vi "Chrg_Dschrg_nodaq.vi"(3 "PS type":enum16{"NHR", "ITECH"}(ring), 4 "PS VISA in":refnum<visa-resource-name>, 5 "PS error in":errorcluster caption="PS error in (no error)", 6 "CyclePath":path=path "C:/Users/ga11/Desktop/VI/results/3PtestCharge.lvm" caption="Filename", 7 "Battery Type":enum16{"30Q", "40T"}(ring), 8 "Charge/discharge":enum8{"Charge", "Discharge"}(ring), 9 "Charge/Discharge Voltage Setpoint":dbl format="%#.6g", 11 "Current Setpoint":dbl format="%#.6g", 13 "Current Cutoff":dbl) -> (14 "PS VISA out":refnum<visa-resource-name>, 19 "PS error out":errorcluster)   [LabVIEW 2020]
uses:
  Drivers-Essentials/Read (Ave Current).vi
  Drivers-NHR-9200/NHR/Public/Data/Low Level/Fetch (Ave Voltage).vi
  <vilib>/Utility/TradDaqScaling.llb/Convert Strain Gauge Reading (scaler).vi
  Drivers-Essentials/NH Research Regenerative Test Series.lvlib
  Drivers-IT-M3400/IT-M3400.lvlib
panel:
  out "StrainGauge":dbl format="%.10f"
  out "Thermocouple":dbl format="%.2f"
  out "Read Ave Current (A)":dbl
  out "Read Ave Voltage (V)":dbl
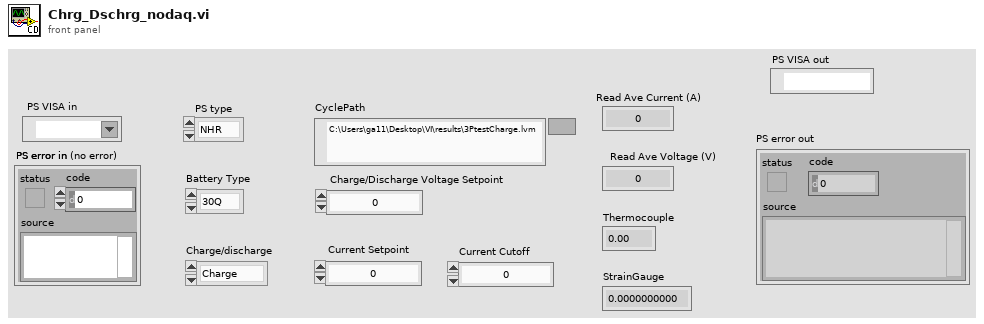
[diagram p1: front panel]
types:
  T1 = cluster{"Voltage Enabled":bool, "Current Enabled":bool, "Power Enabled":bool, "Resistance Enabled":bool}
  T2 = cluster{"Baud Rate":u32, "Parity":u16, "Data Bits":u16, "Stop Bits":u16, "Flow Control":u16}
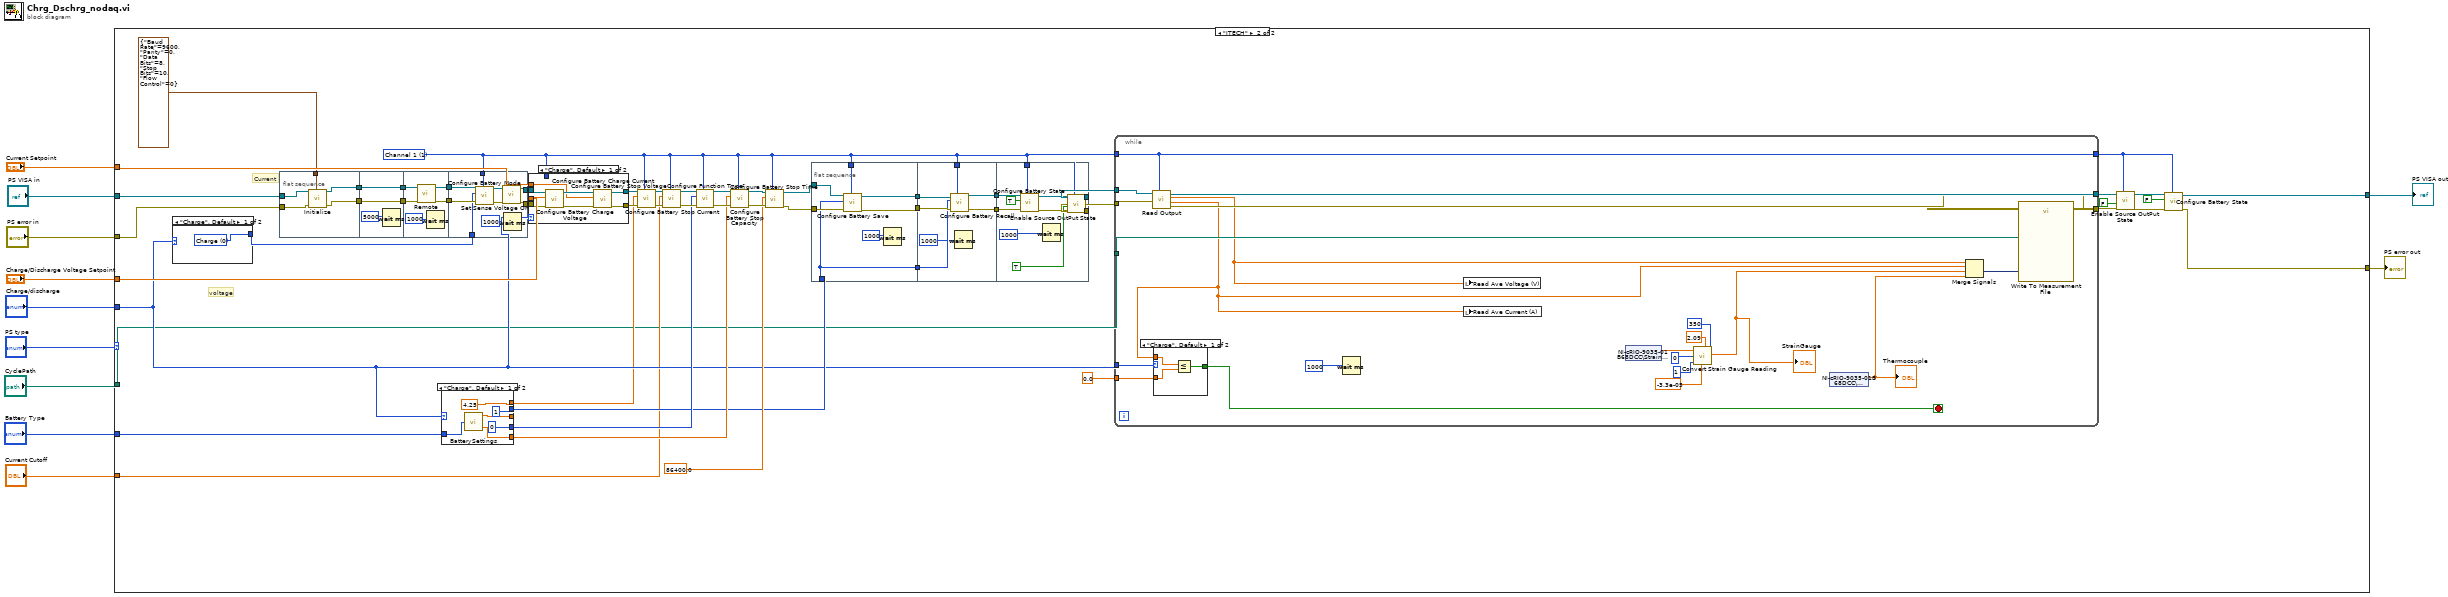
[diagram p0: block diagram]
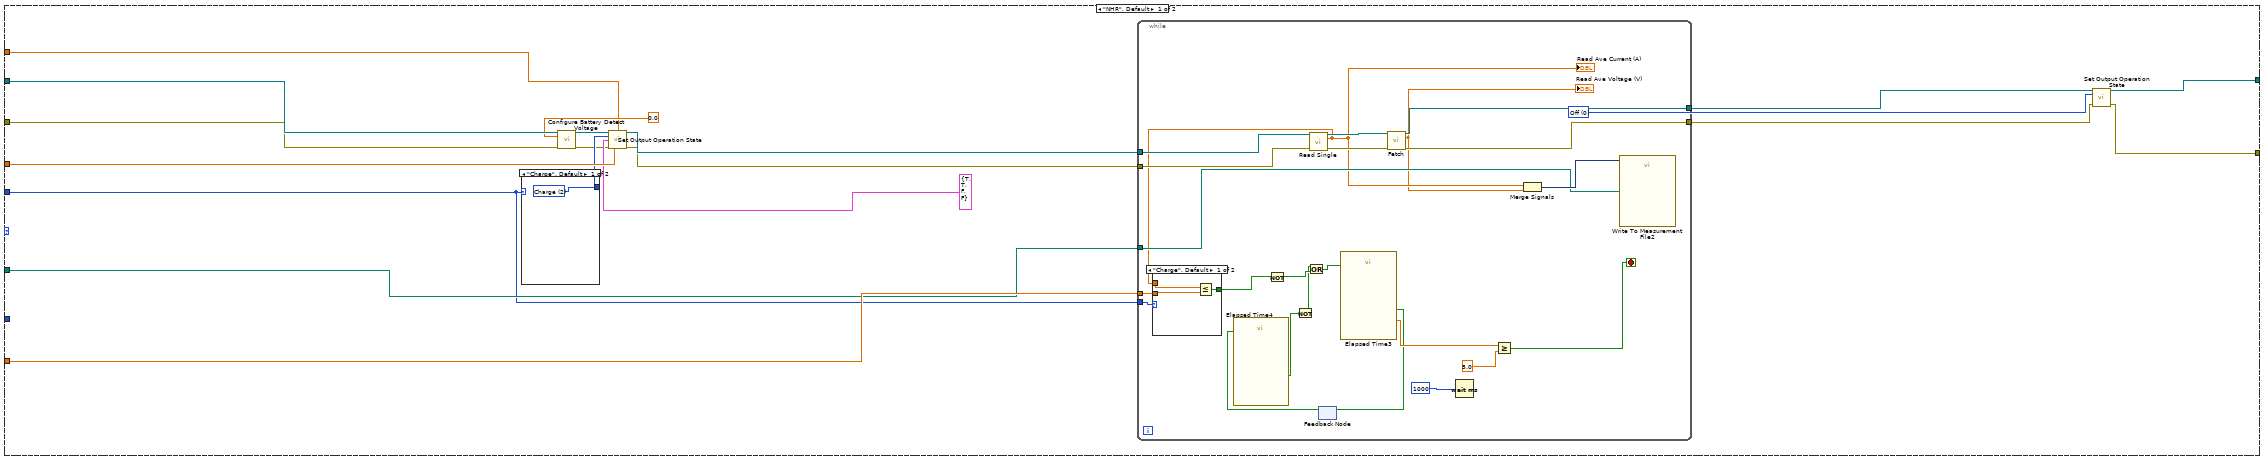
[diagram p2: hidden frame]
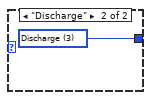
[diagram p3: hidden frame]
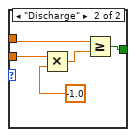
[diagram p4: hidden frame]
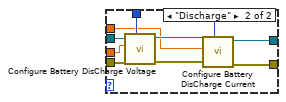
[diagram p5: hidden frame]
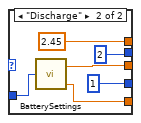
[diagram p6: hidden frame]
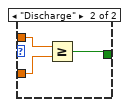
[diagram p7: hidden frame]
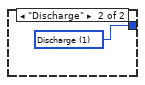
[diagram p8: hidden frame]
diagram:
  n1 = case shown="\"ITECH\"" "PS type" {
    tunnel: "Charge/Discharge Voltage Setpoint" -> [w30 w101]
    tunnel: "Current Setpoint" -> [w12 w99]
    tunnel: "Current Cutoff" -> [w27 w69]
    tunnel: "CyclePath" -> [w24 w67]
    tunnel: "PS VISA in" -> [w20 w80]
    tunnel: "PS error in" -> [w19 w79]
    tunnel: [w17 w66] -> w1
    tunnel: [w16 w100] -> w5
    tunnel: "Charge/discharge" -> [w13 w70]
    tunnel: "Battery Type" -> [_ w98]
    frame "NHR", Default {
      w23 = 0 items=["Off", "Standby", "Charge", "Discharge", "Battery"] ("Mode (0: Off)")
      n2 = case shown="\"Charge\", Default" w13 {
        tunnel: [w31 w32] -> w25
        frame "Charge", Default {
          w31 = 2 items=["Off", "Standby", "Charge", "Discharge", "Battery"] ("Mode (0: Off)")
        }
        frame "Discharge" {
          w32 = 3 items=["Off", "Standby", "Charge", "Discharge", "Battery"] ("Mode (0: Off)")
        }
      }
      n3 = call "Configure Battery Detect Voltage.vi"("VISA resource name"=w20, "Battery Detect Voltage (0V)"=0.0, "error in (no error)"=w19) -> ("VISA resource name out"=w22:refnum<visa-resource-name>, "error out"=w21:errorcluster)  [unwired: 11 in]
      n4 = call "Set Output Operation State.vi"("VISA resource name"=w22, "Voltage Setpoint (0 V)"=w30, "Current Setpoint (0 A)"=w12, "Mode (0: Off)"=w25, "Enable"=T1 {"Voltage Enabled"=TRUE, "Current Enabled"=TRUE, "Power Enabled"=FALSE, "Resistance Enabled"=FALSE}, "error in (no error)"=w21) -> ("VISA resource name out"=w29:refnum<visa-resource-name>, "error out"=w28:errorcluster)  [unwired: 8 in]
      n5 = while {
        tunnel: w29 -> [w53]
        tunnel: w28 -> [w52]
        tunnel: w27 -> [w37]
        tunnel: w24 -> [w40]
        tunnel: [w39] -> w15
        tunnel: [w38] -> w14
        tunnel: w13 -> [w36]
        stop <- w43 stop-if-true
        n6 = call-poly "Read Single.vi"("VISA resource name"=w53, "error in (no error)"=w52) -> ("VISA resource name out"=w54:refnum<visa-resource-name>, "Ave Current (A)"=w35:dbl, "error out"=w55:errorcluster)  [unwired: 11 in]
        "Read Ave Current (A)" <- w35
        n7 = case shown="\"Charge\", Default" w36 {
          tunnel: w37 -> [w57 w62]
          tunnel: w35 -> [w58 w60]
          tunnel: [w56 w59] -> w34
          frame "Charge", Default {
            n8 = Less Or Equal?(x=w58, y=w57) -> (x <= y?=w56:bool)
          }
          frame "Discharge" {
            n9 = Multiply(x=w62, y=-1.0) -> (x*y=w61:dbl)
            n10 = Greater Or Equal?(x=w60, y=w61) -> (x >= y?=w59:bool)
          }
        }
        n11 = Not(x=w34) -> (.not. x?=w49:bool)
        n12 = feedback #1() -> (w41:bool)  [unwired: 1 in]
        n13 = call "Elapsed Time4"("Reset"=w41) -> ("Time has Elapsed"=w48:bool)  [unwired: 11 in, 7 out]
        n14 = Not(x=w48) -> (.not. x?=w47:bool)
        n15 = Or(x=w47, y=w49) -> (x .or. y?=w46:bool)
        n16 = call "Elapsed Time3"("Reset"=w46) -> ("Elapsed Time (s)"=w45:dbl, "Time has Elapsed"=w42:bool)  [unwired: 11 in, 6 out]
        n17 = feedback-in #1(w42) -> ()
        n18 = call-poly "Fetch.vi"("VISA resource name"=w54, "error in (no error)"=w55) -> ("VISA resource name out"=w39:refnum<visa-resource-name>, "Ave Voltage (V)"=w33:dbl, "error out"=w38:errorcluster)  [unwired: 11 in]
        "Read Ave Voltage (V)" <- w33
        n19 = Wait (ms)(milliseconds to wait=1000) -> ()  [unwired: 1 out]
        n20 = Greater Or Equal?(x=w45, y=5.0) -> (x >= y?=w43:bool)
        n21 = Merge Signals "Merge Signals"(w35, w33) -> (w51:dynamicdata)
        n22 = call "Write To Measurement File2"("Signals"=w51, "Filename"=w40) -> ()  [unwired: 15 in, 3 out]
      }
      n23 = call "Set Output Operation State.vi"("VISA resource name"=w15, "Mode (0: Off)"=w23, "error in (no error)"=w14) -> ("VISA resource name out"=w17:refnum<visa-resource-name>, "error out"=w16:errorcluster)  [unwired: 11 in]
    }
    frame "ITECH" {
      w72 = 1 items=["Channel 1"=1, "Channel 2"=2, "Channel 3"=3, "Channel 4"=4, "Channel 5"=5, "Channel 6"=6, "Channel 7"=7, "Channel 8"=8, "Channel 8"=9, "Channel 10"=10, "Channel 11"=11, "Channel 12"=12, "Channel 13"=13, "Channel 14"=14, "Channel 15"=15, "Channel 16"=16] ("Channel")
      # "voltage"
      # "Current"
      n24 = case shown="\"Charge\", Default" w70 {
        tunnel: [w219 w220] -> w86
        frame "Charge", Default {
          w219 = u8 0 items=["Charge", "Discharge"] ("Battery Mode")
        }
        frame "Discharge" {
          w220 = u8 1 items=["Charge", "Discharge"] ("Battery Mode")
        }
      }
      n25 = flat-sequence {
        tunnel: [w117] -> w84
        tunnel: [w118] -> w82
        tunnel: T2 {"Baud Rate"=9600, "Parity"=0, "Data Bits"=8, "Stop Bits"=10, "Flow Control"=0} ("Serial Configuration") -> [w121]
        tunnel: w79 -> [w120]
        tunnel: w80 -> [w119]
        tunnel: w84 -> [w124]
        tunnel: [w124] -> w83
        tunnel: w82 -> [w123]
        tunnel: [w123] -> w81
        tunnel: [w129] -> w88
        tunnel: [w128] -> w87
        tunnel: w83 -> [w127]
        tunnel: w81 -> [w126]
        tunnel: w88 -> [w135]
        tunnel: w87 -> [w137]
        tunnel: w72 -> [w138]
        tunnel: w86 -> [w136]
        tunnel: [w131] -> w65
        tunnel: [w130] -> w64
        frame #0 {
          n26 = call "Initialize.vi"("Serial Configuration"=w121, "error in"=w120, "VISA resource name"=w119) -> ("error out"=w118:errorcluster, "VISA resource name out"=w117:refnum<visa-resource-name>)  [unwired: 7 in]
        }
        frame #1 {
          n27 = Wait (ms)(milliseconds to wait=5000) -> ()  [unwired: 1 out]
        }
        frame #2 {
          n28 = call "Remote.vi"("error in"=w126, "VISA resource name"=w127) -> ("error out"=w128:errorcluster, "VISA resource name out"=w129:refnum<visa-resource-name>)  [unwired: 8 in]
          n29 = Wait (ms)(milliseconds to wait=1000) -> ()  [unwired: 1 out]
        }
        frame #3 {
          n30 = call "Configure Battery Mode.vi"("Channel"=w138, "error in"=w137, "Battery Mode"=w136, "VISA resource name"=w135) -> ("error out"=w132:errorcluster, "VISA resource name out"=w133:refnum<visa-resource-name>)  [unwired: 6 in]
          n31 = call "Set Sense Voltage On.vi"("error in"=w132, "VISA resource name"=w133) -> ("error out"=w131:errorcluster, "VISA resource name out"=w130:refnum<visa-resource-name>)  [unwired: 8 in]
          n32 = Wait (ms)(milliseconds to wait=1000) -> ()  [unwired: 1 out]
        }
      }
      n33 = case shown="\"Charge\", Default" w70 {
        tunnel: w98 -> [w185 w191]
        tunnel: [w184 w189] -> _
        tunnel: [u8 0 ("File") u8 1 ("File")] -> w74
        tunnel: [u8 1 ("File") u8 2 ("File")] -> w71
        tunnel: [w181 w187] -> w73
        tunnel: [4.25 2.45] -> w68
        frame "Charge", Default {
          n34 = call "BatterySettings.vi"("Battery Type"=w185) -> ("RatedCapacity (Ah)"=w181:dbl, "Max Voltage (V)"=w184:dbl)  [unwired: 2 in, 1 out]
        }
        frame "Discharge" {
          n35 = call "BatterySettings.vi"("Battery Type"=w191) -> ("RatedCapacity (Ah)"=w187:dbl, "Min Voltage (V)"=w189:dbl)  [unwired: 2 in, 1 out]
        }
      }
      n36 = case shown="\"Charge\", Default" w70 {
        tunnel: w64 -> [w170 w179]
        tunnel: w65 -> [w169 w178]
        tunnel: [w164 w175] -> w108
        tunnel: [w163 w174] -> w107
        tunnel: w72 -> [_ w173]
        tunnel: w101 -> [w166 w172]
        tunnel: w99 -> [w165 w171]
        frame "Charge", Default {
          n37 = call "Configure Battery Charge Voltage.vi"("error in"=w169, "Charge Voltage(V)"=w166, "VISA resource name"=w170) -> ("error out"=w167:errorcluster, "VISA resource name out"=w168:refnum<visa-resource-name>)  [unwired: 6 in]
          n38 = call "Configure Battery Charge Current.vi"("error in"=w167, "Charge Current(A)"=w165, "VISA resource name"=w168) -> ("error out"=w163:errorcluster, "VISA resource name out"=w164:refnum<visa-resource-name>)  [unwired: 7 in]
        }
        frame "Discharge" {
          n39 = call "Configure Battery DisCharge Voltage.vi"("Channel"=w173, "error in"=w178, "Discharge Voltage(V)"=w172, "VISA resource name"=w179) -> ("error out"=w176:errorcluster, "VISA resource name out"=w177:refnum<visa-resource-name>)  [unwired: 6 in]
          n40 = call "Configure Battery DisCharge Current.vi"("Channel"=w173, "error in"=w176, "Discharge Current(A)"=w171, "VISA resource name"=w177) -> ("error out"=w174:errorcluster, "VISA resource name out"=w175:refnum<visa-resource-name>)  [unwired: 6 in]
        }
      }
      n41 = call "Configure Battery Stop Voltage.vi"("Channel"=w72, "error in"=w107, "Stop Voltage(V)"=w68, "VISA resource name"=w108) -> ("error out"=w115:errorcluster, "VISA resource name out"=w116:refnum<visa-resource-name>)  [unwired: 6 in]
      n42 = call "Configure Battery Stop Current.vi"("Channel"=w72, "error in"=w115, "Stop Current(A)"=w69, "VISA resource name"=w116) -> ("error out"=w76:errorcluster, "VISA resource name out"=w78:refnum<visa-resource-name>)  [unwired: 6 in]
      n43 = call "Configure Function Type.vi"("Channel"=w72, "error in"=w76, "Function Type"=w74, "VISA resource name"=w78) -> ("error out"=w75:errorcluster, "VISA resource name out"=w77:refnum<visa-resource-name>)  [unwired: 6 in]
      n44 = call "Configure Battery Stop Capacity.vi"("Channel"=w72, "error in"=w75, "Stop Capacity(Ah)"=w73, "VISA resource name"=w77) -> ("error out"=w113:errorcluster, "VISA resource name out"=w114:refnum<visa-resource-name>)  [unwired: 6 in]
      n45 = call "Configure Battery Stop Time.vi"("Channel"=w72, "error in"=w113, "Stop Time(S)"=86400.0, "VISA resource name"=w114) -> ("error out"=w90:errorcluster, "VISA resource name out"=w89:refnum<visa-resource-name>)  [unwired: 6 in]
      n46 = flat-sequence {
        tunnel: w71 -> [w144]
        tunnel: w72 -> [w139]
        tunnel: [w142] -> w93
        tunnel: [w144] -> w92
        tunnel: [w141] -> w91
        tunnel: w90 -> [w145]
        tunnel: w89 -> [w143]
        tunnel: [w148] -> w95
        tunnel: [w149] -> w94
        tunnel: w93 -> [w152]
        tunnel: w92 -> [w151]
        tunnel: w91 -> [w150]
        tunnel: w72 -> [w146]
        tunnel: [w156] -> w106
        tunnel: [w155] -> w105
        tunnel: w72 -> [w154]
        tunnel: w95 -> [w162]
        tunnel: w94 -> [w161]
        frame #0 {
          n47 = call "Configure Battery Save.vi"("Channel"=w139, "error in"=w145, "File"=w144, "VISA resource name"=w143) -> ("error out"=w142:errorcluster, "VISA resource name out"=w141:refnum<visa-resource-name>)  [unwired: 6 in]
          n48 = Wait (ms)(milliseconds to wait=1000) -> ()  [unwired: 1 out]
        }
        frame #1 {
          n49 = call "Configure Battery Recall.vi"("Channel"=w146, "error in"=w152, "File"=w151, "VISA resource name"=w150) -> ("error out"=w149:errorcluster, "VISA resource name out"=w148:refnum<visa-resource-name>)  [unwired: 6 in]
          n50 = Wait (ms)(milliseconds to wait=1000) -> ()  [unwired: 1 out]
        }
        frame #2 {
          n51 = call "Configure Battery State.vi"("Channel"=w154, "error in"=w161, "State"=TRUE, "VISA resource name"=w162) -> ("error out"=w159:errorcluster, "VISA resource name out"=w160:refnum<visa-resource-name>)  [unwired: 6 in]
          n52 = Wait (ms)(milliseconds to wait=1000) -> ()  [unwired: 1 out]
          n53 = call "Enable Source OutPut State.vi"("Channel"=w154, "error in"=w159, "State"=TRUE ("Enable Output|Intput"), "VISA resource name"=w160) -> ("error out"=w155:errorcluster, "VISA resource name out"=w156:refnum<visa-resource-name>)  [unwired: 6 in]
        }
      }
      n54 = while {
        tunnel: [w204] -> w104
        tunnel: [w197] -> w103
        tunnel: w106 -> [w212]
        tunnel: w105 -> [w211]
        tunnel: w72 -> [w203]
        tunnel: [w203] -> w102
        tunnel: w67 -> [w209]
        tunnel: 0.0 -> [w207]
        tunnel: w70 -> [w205]
        stop <- w206 stop-if-true
        n55 = call "Read Output.vi"("Channel"=w203, "error in"=w211, "VISA resource name"=w212) -> ("error out"=w197:errorcluster, "Read Current(A)"=w195:dbl, "Read Voltage(V)"=w196:dbl, "VISA resource name out"=w204:refnum<visa-resource-name>)  [unwired: 5 in]
        n56 = case shown="\"Charge\", Default" w205 {
          tunnel: w207 -> [w214 w217]
          tunnel: w195 -> [w215 w218]
          tunnel: [w213 w216] -> w206
          frame "Charge", Default {
            n57 = Less Or Equal?(x=w215, y=w214) -> (x <= y?=w213:bool)
          }
          frame "Discharge" {
            n58 = Greater Or Equal?(x=w218, y=w217) -> (x >= y?=w216:bool)
          }
        }
        n59 = Wait (ms)(milliseconds to wait=1000) -> ()  [unwired: 1 out]
        n60 = local write "Read Ave Voltage (V)"(w196) -> ()
        n61 = local write "Read Ave Current (A)"(w195) -> ()
        n62 = shared-variable "NI-cRIO-9035-01B68DCC\\Strain Gauge\\AI0"() -> (w192:dbl)  [unwired: 1 in, 1 out]
        n63 = call-poly <vilib>:"Convert Strain Gauge Reading.vi"("Vsg (0.0)"=w192, "Bridge Configuration\n(3:Half Bridge II)"=0, "Vex (3.33)"=1, "Vinit (0.0)"=-3.3e-05, "GF (2.0)"=2.09, "Rg (120)"=350) -> ("Strain"=w194:sgl)  [unwired: 4 in]
        "StrainGauge" <- w194
        n64 = shared-variable "NI-cRIO-9035-01B68DCC\\Thermocouple\\CH0"() -> (w193:dbl)  [unwired: 1 in, 1 out]
        "Thermocouple" <- w193
        n65 = Merge Signals "Merge Signals"(w196, w195, w194, w193) -> (w210:dynamicdata)
        n66 = call "Write To Measurement File"("Signals"=w210, "Filename"=w209) -> ()  [unwired: 15 in, 3 out]
      }
      n67 = call "Enable Source OutPut State.vi"("Channel"=w102, "error in"=w103, "State"=FALSE, "VISA resource name"=w104) -> ("error out"=w111:errorcluster, "VISA resource name out"=w112:refnum<visa-resource-name>)  [unwired: 6 in]
      n68 = call "Configure Battery State.vi"("Channel"=w102, "error in"=w111, "State"=FALSE, "VISA resource name"=w112) -> ("error out"=w100:errorcluster, "VISA resource name out"=w66:refnum<visa-resource-name>)  [unwired: 6 in]
    }
  }
  "PS error out" <- w5
  "PS VISA out" <- w1
